vi "VisionMain.vi"   [LabVIEW 2018]
uses:
  Vision Data.ctl
  Vision Global.vi
  <vilib>/Rock Robotics/Network Tables/NT Read Number.vi
types:
  T1 = typedef "Vision Data.ctl" = cluster{"xOffset":dbl, "yOffset":dbl, "area":dbl, "skewOffset":dbl, "hasTarget":dbl}
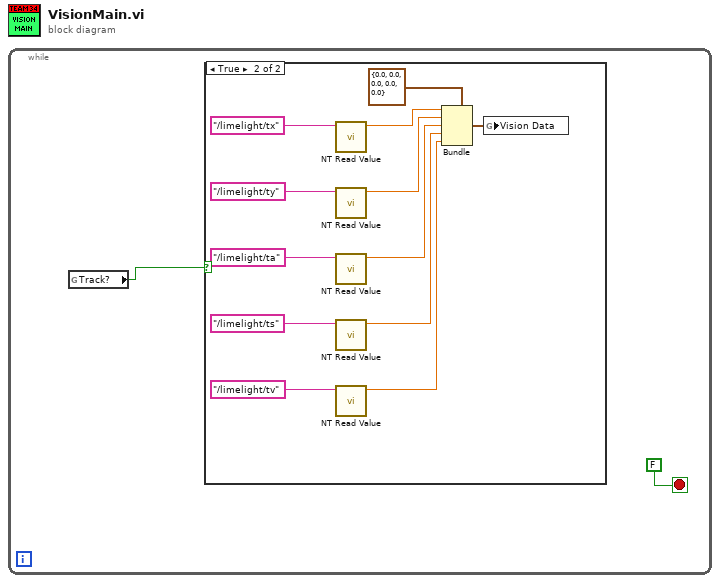
[diagram p0: block diagram]
diagram:
  n1 = while {
    stop <- FALSE stop-if-true
    n2 = global read "Vision Global.vi" "Track?"() -> (w1:bool)
    n3 = case shown="True" w1 {
      frame False {
      }
      frame True {
        n4 = call-poly <vilib>:"NT Read Value.vi"("Name"="/limelight/tx") -> ("Numeric"=w10:dbl)  [unwired: 9 in, 1 out]
        n5 = call-poly <vilib>:"NT Read Value.vi"("Name"="/limelight/ty") -> ("Numeric"=w9:dbl)  [unwired: 9 in, 1 out]
        n6 = call-poly <vilib>:"NT Read Value.vi"("Name"="/limelight/ta") -> ("Numeric"=w13:dbl)  [unwired: 9 in, 1 out]
        n7 = call-poly <vilib>:"NT Read Value.vi"("Name"="/limelight/ts") -> ("Numeric"=w12:dbl)  [unwired: 9 in, 1 out]
        n8 = call-poly <vilib>:"NT Read Value.vi"("Name"="/limelight/tv") -> ("Numeric"=w11:dbl)  [unwired: 9 in, 1 out]
        n9 = Bundle(cluster=T1 {"xOffset"=0.0, "yOffset"=0.0, "area"=0.0, "skewOffset"=0.0, "hasTarget"=0.0} ("Vision Data"), "xOffset"=w10, "yOffset"=w9, "area"=w13, "skewOffset"=w12, "hasTarget"=w11) -> (w14:T1)
        n10 = global write "Vision Global.vi" "Vision Data"(w14) -> ()
      }
    }
  }
